vi "MomentOfReplacementPasseTest.vi"(9 "Replace active":bool, 10 "IA State Input":T1) -> (1 "Number of goals":i16, 2 "Time to replace?":bool)   [LabVIEW 2017]
uses:
  Core/AI Input.ctl
  Core/AI Robot.ctl
  Intel/Functions Enum.ctl
  Intel/AttackerStates.ctl
  Path Planning/RRT/PathDests.ctl
  Path Planning/RRT/PathDest.ctl
  Core/AI Ball.ctl
  Core/Field Size.ctl
  Core/AI Judge.ctl
  Intel/Command Enum.ctl
  Util/Events/Events.ctl
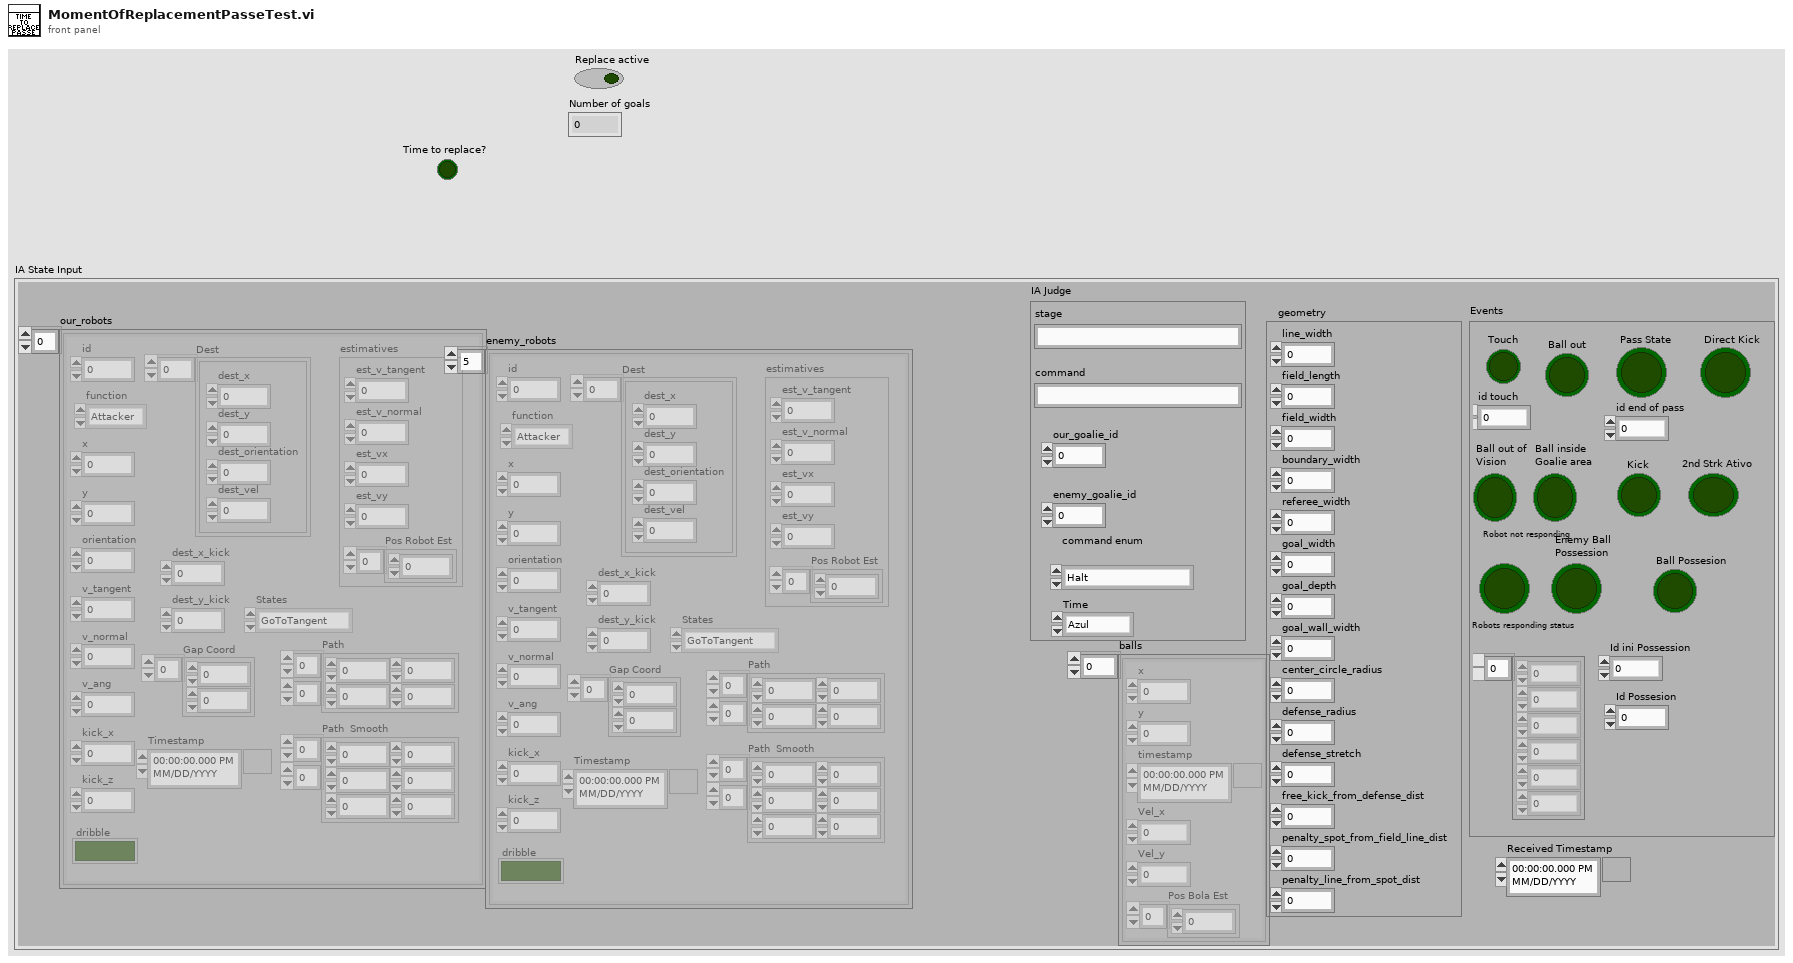
[diagram p1: front panel]
types:
  T1 = typedef "AI Input.ctl" = cluster{"our_robots":T2[], "enemy_robots":T2[], "balls":T7[], "geometry":T8, "IA Judge":T9, "Received Timestamp":timestamp, "Events":T11}
  T2 = typedef "AI Robot.ctl" = cluster{"id":u32, "function":T3, "x":dbl, "y":dbl, "orientation":dbl, "v_tangent":dbl, "v_normal":dbl, "v_ang":dbl, "kick_x":dbl, "kick_z":dbl, "dribble":bool, "Timestamp":timestamp, "estimatives":cluster{"est_v_tangent":dbl, "est_v_normal":dbl, "est_vx":dbl, "est_vy":dbl, "Pos Robot Est":dbl[]}, "dest_x_kick":dbl, "dest_y_kick":dbl, "Gap Coord":dbl[], "States":T4, "Path ":dbl[][], "Path  Smooth":dbl[][], "Dest":T5}
  T3 = typedef "Functions Enum.ctl" = enum16{"2nd Striker", "Attacker", "Goalie", "Defender", "Striker", "Goto 0", "Dummy", "Kicker", "ZigZag 0", "ZigZag 1", "ZigZag 2", "ZigZag 3", "ZigZag 4", "ZigZag 5", "ZigZag 6", "ZigZag 7", "ZigZag 8", ""}
  T4 = typedef "AttackerStates.ctl" = enum16{"Pass", "GoToTangent", "BallGetting", "GoToKick", ""}
  T5 = typedef "PathDests.ctl" = T6[]
  T6 = typedef "PathDest.ctl" = cluster{"dest_x":dbl, "dest_y":dbl, "dest_orientation":dbl, "dest_vel":dbl}
  T7 = typedef "AI Ball.ctl" = cluster{"x":dbl, "y":dbl, "timestamp":timestamp, "Vel_x":dbl, "Vel_y":dbl, "Pos Bola Est":dbl[]}
  T8 = typedef "Field Size.ctl" = cluster{"line_width":u32, "field_length":u32, "field_width":u32, "boundary_width":u32, "referee_width":u32, "goal_width":u32, "goal_depth":u32, "goal_wall_width":u32, "center_circle_radius":u32, "defense_radius":u32, "defense_stretch":u32, "free_kick_from_defense_dist":u32, "penalty_spot_from_field_line_dist":u32, "penalty_line_from_spot_dist":u32}
  T9 = typedef "AI Judge.ctl" = cluster{"stage":string, "command":string, "our_goalie_id":dbl, "enemy_goalie_id":dbl, "command enum":T10, "Time":enum16{"Azul", "Amarelo"}}
  T10 = typedef "Command Enum.ctl" = enum16{"Halt", "Stop", "Force Start", "PKA Normal Start", "Prepare Kickoff Ally", "PKE Normal Start", "Prepare Kickoff Enemy", "Prepare Penalty Ally", "PPA Normal Start", "Prepare Penalty Enemy", "PPE Normal Start", "Direct Free Enemy", "Direct Free Ally", "Indirect Free Enemy", "Indirect Free Ally", "Timeout Enemy", "Timeout Ally", "Goal Enemy", "Goal Ally", "Ball Placement Enemy", "Ball Placement Ally", "Normal Half Time", "Extra Time Break", "Extra Half Time", "None", "Post Game"}
  T11 = typedef "Events.ctl" = cluster{"Touch":bool, "Ball out":bool, "id touch":dbl, "Ball out of \nVision":bool, "Ball inside \nGoalie area":bool, "Robot not responding":bool, "Robots responding status":dbl[], "Enemy Ball \nPossession":bool, "Pass State":bool, "id end of pass":dbl, "Kick":bool, "Id ini Possession":dbl, "Ball Possesion":bool, "Id Possesion":dbl, "Direct Kick":bool, "2nd Strk Ativo":bool}
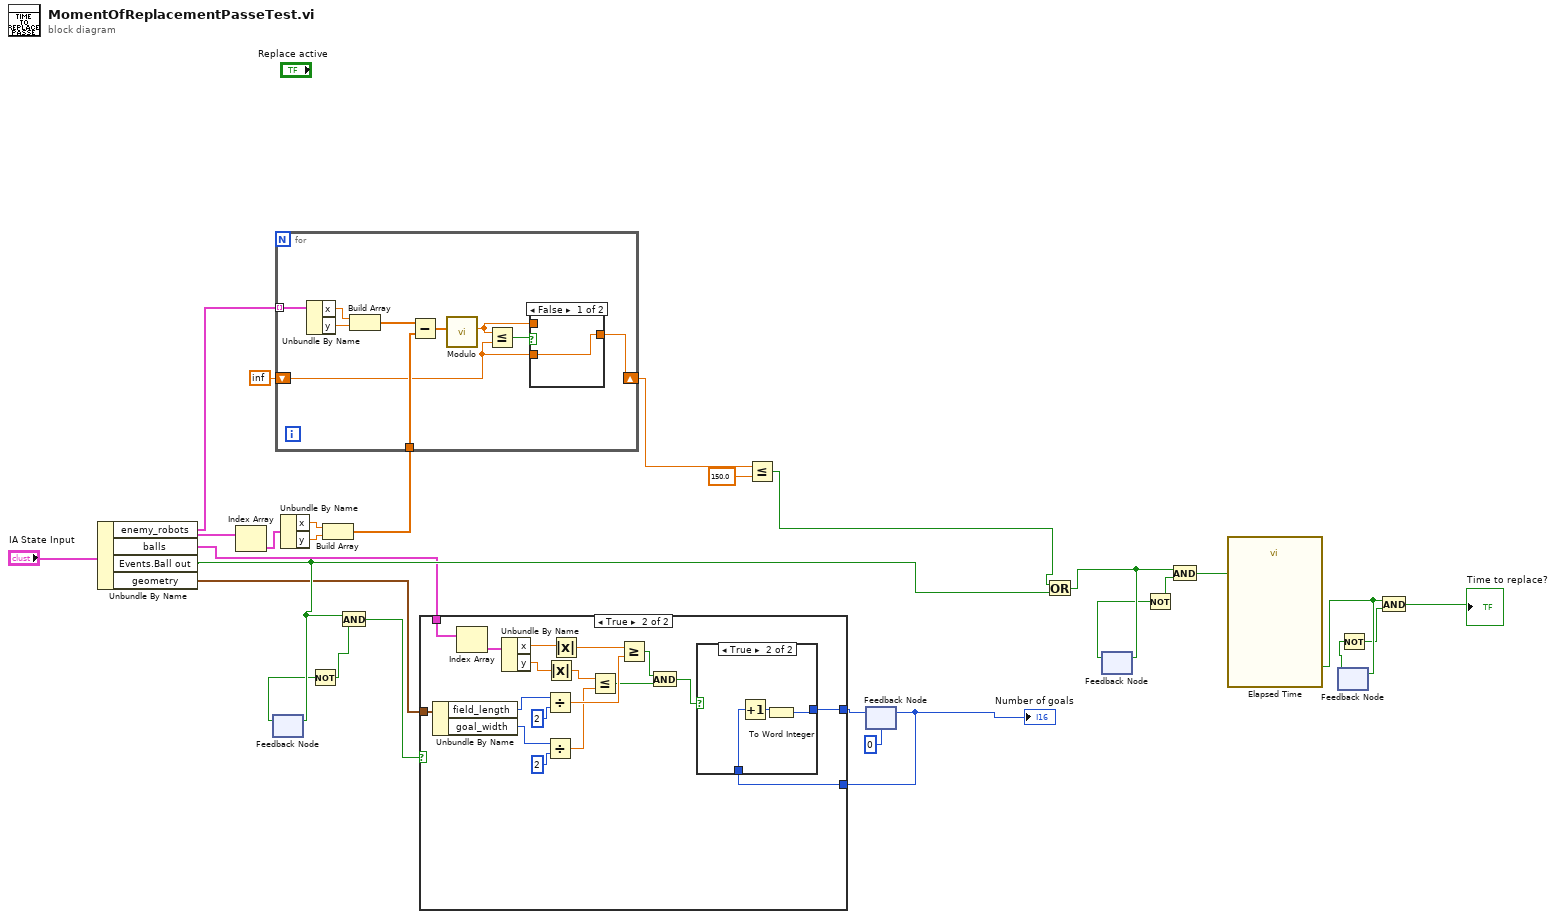
[diagram p0: block diagram]
diagram:
  n1 = Unbundle By Name("IA State Input") -> ("enemy_robots"=w26:T2[], "balls"=w13:T7[], "Events.Ball out"=w16:bool, "geometry"=w12:T8)
  n2 = Index Array(array=w13) -> (element=w25:T7)  [unwired: 1 in]
  n3 = feedback #1() -> (w15:bool)  [unwired: 1 in]
  n4 = feedback-in #1(w16) -> ()
  n5 = Unbundle By Name(w25) -> ("x"=w24:dbl, "y"=w23:dbl)
  n6 = Not(x=w15) -> (.not. x?=w17:bool)
  n7 = Build Array(w24, w23) -> (w22:dbl[])
  n8 = for {
    tunnel: w26 -> [w37] mode=indexing
    tunnel: w22 -> [w33]
    shift-right: [w30] -> w20
    shift-left: inf ("Modulo") -> [w28]
    n9 = Unbundle By Name(w37) -> ("x"=w36:dbl, "y"=w35:dbl)
    n10 = Build Array(w36, w35) -> (w34:dbl[])
    n11 = Subtract(x=w34, y=w33) -> (x-y=w32:dbl[])
    n12 = call "Modulo.vi"("2D vector"=w32) -> ("Modulo"=w29:dbl)  [unwired: 10 in]
    n13 = Less Or Equal?(x=w29, y=w28) -> (x <= y?=w31:bool)
    n14 = case shown="False" w31 {
      tunnel: [w38 w39] -> w30
      tunnel: w29 -> [_ w39]
      tunnel: w28 -> [w38 _]
      frame False {
      }
      frame True {
      }
    }
  }
  n15 = And(x=w16, y=w17) -> (x .and. y?=w14:bool)
  n16 = Less Or Equal?(x=w20, y=150.0) -> (x <= y?=w18:bool)
  n17 = feedback #2(i16 0) -> (w9:i16)
  "Number of goals" <- w9
  n18 = case shown="True" w14 {
    tunnel: w13 -> [_ w58]
    tunnel: w12 -> [_ w53]
    tunnel: [w40 w42] -> w11
    tunnel: w9 -> [w40 w41]
    frame False {
    }
    frame True {
      n19 = Unbundle By Name(w53) -> ("field_length"=w52:u32, "goal_width"=w49:u32)
      n20 = Index Array(array=w58) -> (element=w57:T7)  [unwired: 1 in]
      n21 = Unbundle By Name(w57) -> ("x"=w56:dbl, "y"=w55:dbl)
      n22 = Divide(x=w52, y=u32 2) -> (x/y=w48:dbl)
      n23 = Divide(x=w49, y=u32 2) -> (x/y=w46:dbl)
      n24 = Absolute Value(x=w55) -> (abs(x)=w47:dbl)
      n25 = Absolute Value(x=w56) -> (abs(x)=w54:dbl)
      n26 = Less Or Equal?(x=w47, y=w46) -> (x <= y?=w44:bool)
      n27 = Greater Or Equal?(x=w54, y=w48) -> (x >= y?=w45:bool)
      n28 = And(x=w45, y=w44) -> (x .and. y?=w43:bool)
      n29 = case shown="True" w43 {
        tunnel: [w59 w60] -> w42
        tunnel: w41 -> [w59 w62]
        frame False {
        }
        frame True {
          n30 = Increment(x=w62) -> (x+1=w61:i16)
          n31 = To Word Integer(number=w61) -> (16bit integer=w60:i16)
        }
      }
    }
  }
  n32 = feedback-in #2(w11) -> ()
  n33 = Or(x=w18, y=w16) -> (x .or. y?=w7:bool)
  n34 = feedback #3() -> (w6:bool)  [unwired: 1 in]
  n35 = feedback-in #3(w7) -> ()
  n36 = Not(x=w6) -> (.not. x?=w8:bool)
  n37 = And(x=w7, y=w8) -> (x .and. y?=w5:bool)
  n38 = call "Elapsed Time"("Auto Reset"=w5) -> ("Time has Elapsed"=w4:bool)  [unwired: 11 in, 7 out]
  n39 = feedback #4() -> (w2:bool)  [unwired: 1 in]
  n40 = feedback-in #4(w4) -> ()
  n41 = Not(x=w2) -> (.not. x?=w1:bool)
  n42 = And(x=w4, y=w1) -> (x .and. y?=→"Time to replace?":bool)
